vi "DOS cmd.vi"(8 "错误输入（无错误）":errorcluster) -> (0 "error out":errorcluster caption="错误输出")   [LabVIEW 2016, in "update.lvlib"]
uses:
  update.lvlib
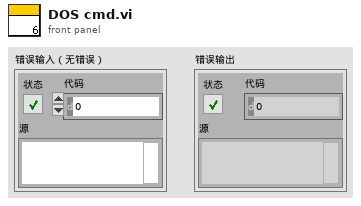
[diagram p1: front panel]
types:
  T1 = enum16{"open", "replace", "create", "open or create", "replace or create", "replace or create with confirmation"}
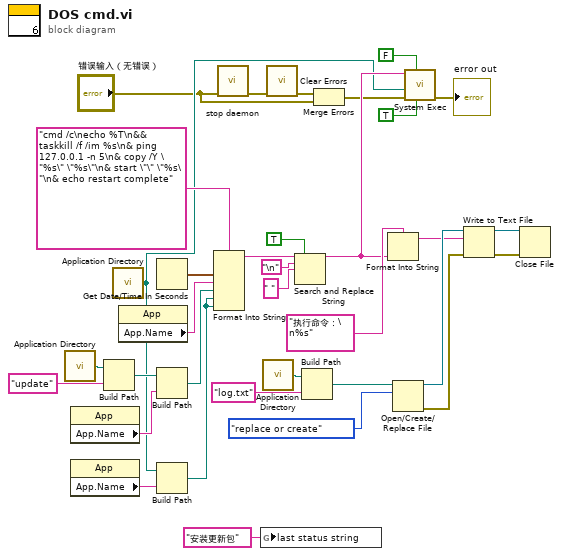
[diagram p0: block diagram]
diagram:
  n1 = call <vilib>:"Application Directory.vi"() -> ("Application Directory"=w23:path)
  n2 = property class="App"() -> ("App.Name"=w20:string)  [unwired: 2 in, 2 out]
  n3 = property class="App"() -> ("App.Name"=w19:string)  [unwired: 2 in, 2 out]
  n4 = Build Path(base path=w23, name or relative path="update" ("名称或相对路径")) -> (appended path=w21:path)
  n5 = call <vilib>:"Application Directory.vi"() -> ("Application Directory"=w6:path)
  n6 = property class="App"() -> ("App.Name"=w7:string)  [unwired: 2 in, 2 out]
  n7 = Get Date/Time In Seconds() -> (seconds since 1Jan1904=w24:timestamp)
  n8 = Build Path(base path=w21, name or relative path=w20) -> (appended path=w18:path)
  n9 = Build Path(base path=w6, name or relative path=w19) -> (appended path=w17:path)
  n10 = Format Into String(format string="cmd /c\necho %T\n&& taskkill /f /im %s\n& ping 127.0.0.1 -n 5\n& copy /Y \"%s\" \"%s\"\n& start \"\" \"%s\"\n& echo restart complete" ("文本"), w24, w7, w18, w17, w17) -> (resulting string=w14:string)  [unwired: 2 in, 1 out]
  n11 = call "stop daemon.vi"("error in (no error)"="错误输入（无错误）") -> ("error out"=w9:errorcluster)  [unwired: 10 in]
  n12 = global write "更新全局变量.vi" "last status string"("安装更新包" ("last status string")) -> ()
  n13 = call <vilib>:"Application Directory.vi"() -> ("Application Directory"=w5:path)
  n14 = call <vilib>:"Clear Errors.vi"("error in (no error)"=w9) -> ("error out"=w4:errorcluster)  [unwired: 5 in, 1 out]
  n15 = Search and Replace String(replace all?=TRUE ("替换全部？(F)"), input string=w14, search string="\n", replace string=" " ("替换字符串(\"\")")) -> (result string=w11:string)  [unwired: 4 in, 3 out]
  n16 = Build Path(base path=w5, name or relative path="log.txt" ("名称或相对路径")) -> (appended path=w29:path)
  n17 = Merge Errors(w4, "错误输入（无错误）") -> (w2:errorcluster)
  n18 = Format Into String(format string="执行命令：\n%s" ("格式字符串"), w11) -> (resulting string=w26:string)  [unwired: 2 in, 1 out]
  n19 = Open/Create/Replace File(file path (use dialog)=w29, operation (0:open)=T1."replace or create" ("操作(0:open)")) -> (refnum out=w31:refnum<file>, error out=w34:errorcluster)  [unwired: 4 in, 1 out]
  n20 = call <vilib>:"System Exec.vi"("run minimized? (F)"=TRUE, "wait until completion? (T)"=FALSE, "error in (no error)"=w2, "working directory"=w6, "command line"=w11) -> ("error out"=→"error out":errorcluster)  [unwired: 3 in, 3 out]
  n21 = Write to Text File(file (use dialog)=w31, text=w26, error in=w34) -> (refnum out=w32:refnum<file>, error out=w33:errorcluster)  [unwired: 1 in, 1 out]
  n22 = Close File(refnum=w32, error in=w33) -> ()  [unwired: 2 out]
